vi "get_enable.vi"(8 "error in (no error)":errorcluster, 11 "system.logging.provider in":refnum<class "system.logging.provider.lvclass">) -> (0 "error out":errorcluster, 2 "enable":bool, 3 "system.logging.provider out":refnum<class "system.logging.provider.lvclass">)   [LabVIEW 2021, in "system.logging.provider.lvclass"]
uses:
  system.logging.provider.lvclass
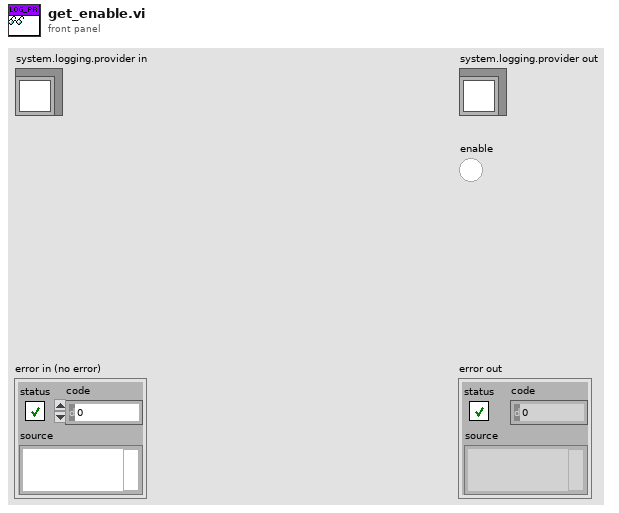
[diagram p1: front panel]
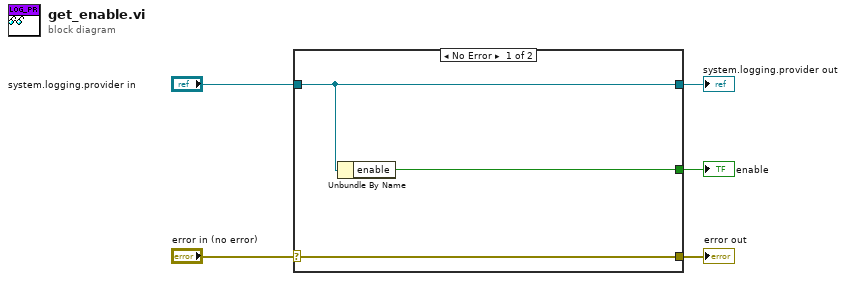
[diagram p0: block diagram]
diagram:
  n1 = case shown="No Error" "error in (no error)" {
    selector: "error in (no error)" -> [w8 w9]
    tunnel: [w8 w9] -> w4
    tunnel: [w7 w10] -> w2
    tunnel: "system.logging.provider in" -> [w7 w10]
    tunnel: [w6 _] -> w1
    frame No Error {
      n2 = Unbundle By Name(w7) -> ("enable"=w6:bool)
    }
    frame Error {
    }
  }
  "error out" <- w4
  "system.logging.provider out" <- w2
  "enable" <- w1
